vi "Gauge Range and Color Set.vi"(8 "Alarm Maximum":dbl, 9 "Nominal Target":dbl, 10 "Alarm Minimum":dbl, 11 "reference":refnum<vi>) -> ()   [LabVIEW 2018]
panel:
  in  "Color Green":u32(colorbox)=32768
  in  "Color Yellow":u32(colorbox)=16776960
  in  "Color Red":u32(colorbox)=16711680
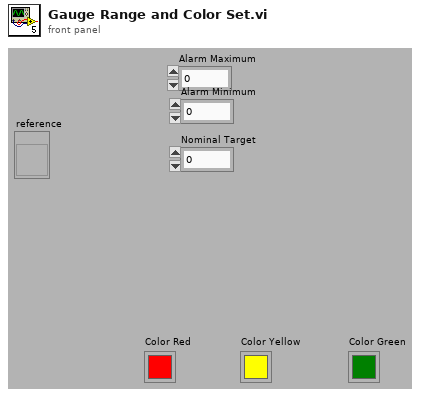
[diagram p1: front panel]
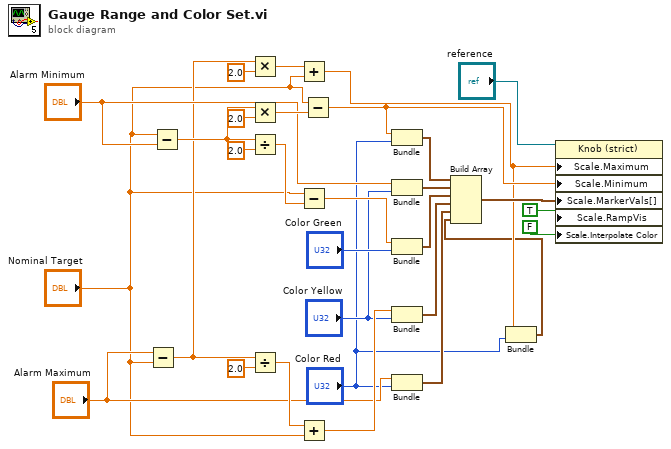
[diagram p0: block diagram]
diagram:
  n1 = Subtract(x="Alarm Maximum", y="Nominal Target") -> (x-y=w16:dbl)
  n2 = Subtract(x="Nominal Target", y="Alarm Minimum") -> (x-y=w24:dbl)
  n3 = Multiply(x=w16, y=2.0) -> (x*y=w27:dbl)
  n4 = Multiply(x=w24, y=2.0) -> (x*y=w29:dbl)
  n5 = Divide(x=w24, y=2.0) -> (x/y=w22:dbl)
  n6 = Divide(x=w16, y=2.0) -> (x/y=w14:dbl)
  n7 = Add(x=w27, y="Nominal Target") -> (x+y=w3:dbl)
  n8 = Subtract(x="Nominal Target", y=w22) -> (x-y=w19:dbl)
  n9 = Add(x=w14, y="Nominal Target") -> (x+y=w13:dbl)
  n10 = Subtract(x="Nominal Target", y=w29) -> (x-y=w26:dbl)
  n11 = Bundle(w26, "Color Red"="Color Red") -> (w25:cluster{dbl, "Color Red":u32})  [unwired: 1 in]
  n12 = Bundle("Alarm Minimum"="Alarm Minimum", "Color Yellow"="Color Yellow") -> (w20:cluster{"Alarm Minimum":dbl, "Color Yellow":u32})  [unwired: 1 in]
  n13 = Bundle(w19, "Color Green"="Color Green") -> (w17:cluster{dbl, "Color Green":u32})  [unwired: 1 in]
  n14 = Bundle(w13, "Color Yellow"="Color Yellow") -> (w11:cluster{dbl, "Color Yellow":u32})  [unwired: 1 in]
  n15 = Bundle("Alarm Maximum"="Alarm Maximum", "Color Red"="Color Red") -> (w9:cluster{"Alarm Maximum":dbl, "Color Red":u32})  [unwired: 1 in]
  n16 = Bundle(w3, "Color Red"="Color Red") -> (w1:cluster{dbl, "Color Red":u32})  [unwired: 1 in]
  n17 = Build Array(w25, w20, w17, w11, w9, w1) -> (w8:cluster{"Alarm Maximum":dbl, "Color Red":u32}[])
  n18 = property class="Knob (strict)"(reference="reference", "Scale.Maximum"=w3, "Scale.Minimum"=w26, "Scale.MarkerVals[]"=w8, "Scale.RampVis"=TRUE ("Scale.Ramp Visible"), "Scale.Interpolate Color"=FALSE) -> ()  [unwired: 1 in, 2 out]
